vi "Definition.vi"(11 "Entity":refnum<class "Entity.lvclass">) -> (2 "Entity Definition":refnum<class "Type.lvclass">[](array[class]))   [LabVIEW 2022 SP3, in "Conditum.lvlib" / "Entity.lvclass"]
uses:
  Entity.lvclass
  Entity.lvclass/Entity.ctl
  Columns/Type/Type.lvclass
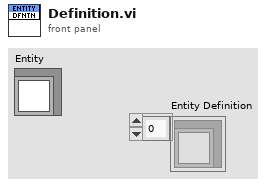
[diagram p1: front panel]
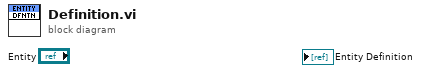
[diagram p0: block diagram]
diagram:
